vi "cluster.vi"() -> ()   [LabVIEW 2019]
panel:
  out "salary":dbl
  out "name":string
  out "agec":dbl
  in  "input  ubn":T1
  in  "c b":dbl
  in  "a":dbl
  out "output cluster":cluster{"a":dbl, "b":dbl}
  in  "input cluster":cluster{"a":dbl, " b":dbl}
  # "bundle by name"
  # "Unbundle by name"
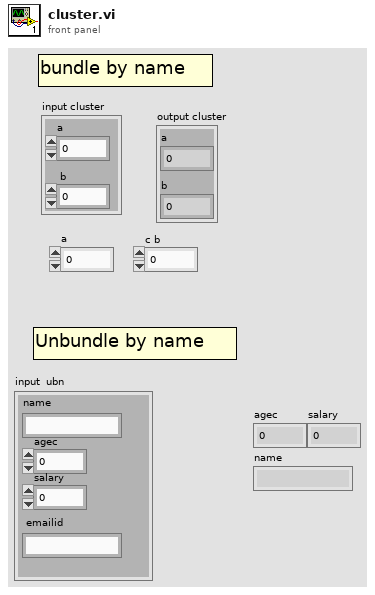
[diagram p1: front panel]
types:
  T1 = cluster{"agec":dbl, "name":string, "salary":dbl, " emailid":string}
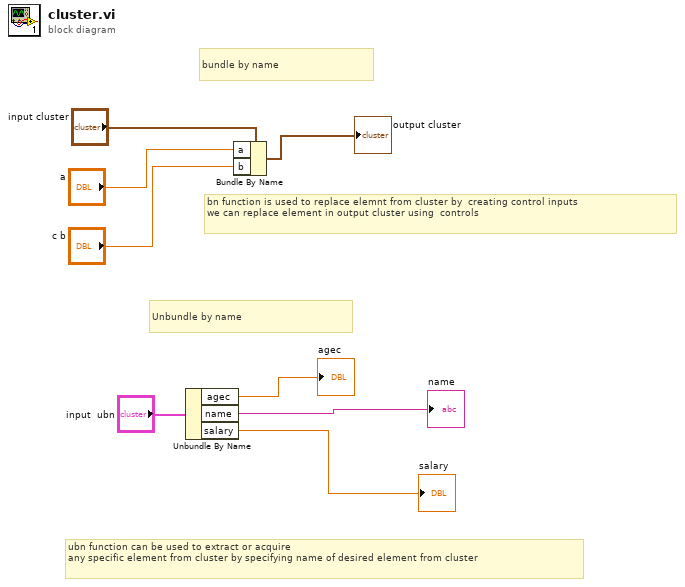
[diagram p0: block diagram]
diagram:
  # "ubn function can be used to extract or acquire \nany specific element from cluster by specifying name of desired element from cluster"
  # "bn function is used to replace elemnt from cluster by  creating control inputs\nwe can replace element in output cluster using  controls"
  # "Unbundle by name"
  # "bundle by name"
  n1 = Unbundle By Name("input  ubn") -> ("agec"=→"agec":dbl, "name"=→"name":string, "salary"=→"salary":dbl)
  n2 = Bundle By Name(cluster="input cluster", "a"="a", "b"="c b") -> (→"output cluster":cluster{"a":dbl, " b":dbl})
